vi "shutDownHW.vi"(8 "error in (no error)":errorcluster, 11 "WindowsTarget in":refnum<class "WindowsTarget.lvclass">) -> (0 "error out":errorcluster, 3 "WindowsTarget out":refnum<class "WindowsTarget.lvclass">)   [LabVIEW 2012, in "WindowsTarget.lvclass"]
doc: "Performs any operations necessary to shut down the hardware."
uses:
  WindowsTarget.lvclass
  Target/Target.lvclass
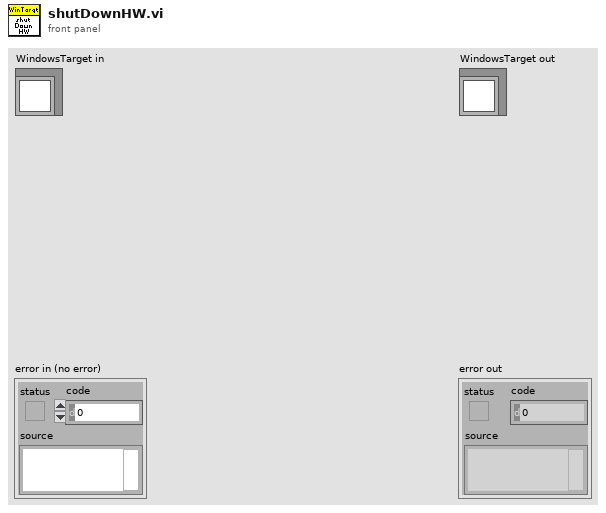
[diagram p1: front panel]
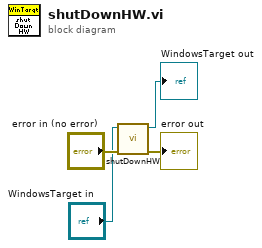
[diagram p0: block diagram]
diagram:
  n1 = call-parent "shutDownHW.vi"("error in (no error)"="error in (no error)", "Target in"="WindowsTarget in") -> ("error out"=→"error out":errorcluster, "Target out"=→"WindowsTarget out":refnum<class "WindowsTarget.lvclass">)  [unwired: 8 in]
